vi "Set extraction scrollbar.vi"(8 "error in (no error)":errorcluster, 10 "Min frame":u32, 11 "Number of frames":u32) -> (0 "error out":errorcluster)   [LabVIEW 2017]
uses:
  Globals/gl_Time series viewer globals.vi
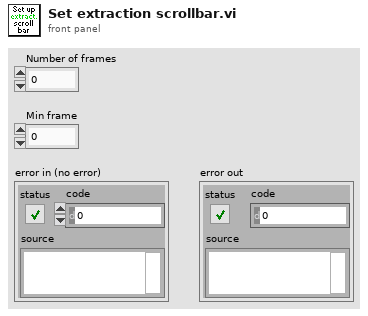
[diagram p1: front panel]
types:
  T1 = typedef "Time series viewer refs.ctl" = cluster{"This VI":refnum<vi>, "Image control":refnum<vi>, "AVI Mode ind":refnum<vi>, "Play":refnum<vi>, "Stop":refnum<vi>, "Back":refnum<vi>, "Scrollbar":refnum<vi>, "Video length info":refnum<vi>, "Expected speed values":refnum<vi>, "Intensity":refnum<vi>, "Path":refnum<vi>, "Selection sliders":refnum<vi>, "Speed Graph ref":refnum<vi>, "Frame rate set (fps)":refnum<vi>, "Channel to load":refnum<vi>, "Number of rows to generate":refnum<vi>, "Colour":refnum<vi>}
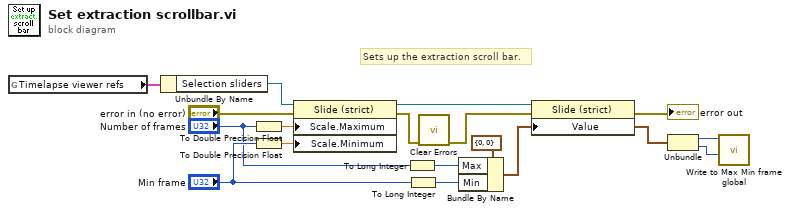
[diagram p0: block diagram]
diagram:
  # "Sets up the extraction scroll bar."
  n1 = global read "gl_Time series viewer globals.vi" "Timelapse viewer refs"() -> (w6:T1)
  n2 = Unbundle By Name(w6) -> ("Selection sliders"=w7:refnum<vi>)
  n3 = To Double Precision Float(number="Number of frames") -> (double precision float=w8:dbl)
  n4 = To Double Precision Float(number="Min frame") -> (double precision float=w16:dbl)
  n5 = property on="Property Node" class="Slide (strict)"(reference=w7, error in="error in (no error)", "Scale.Maximum"=w8, "Scale.Minimum"=w16) -> (reference out=w12:refnum<vi>, error out=w13:errorcluster)
  n6 = To Long Integer(number="Number of frames") -> (32bit integer=w3:i32)
  n7 = To Long Integer(number="Min frame") -> (32bit integer=w2:i32)
  n8 = call <vilib>:"Clear Errors.vi"("error in (no error)"=w13) -> ("error out"=w1:errorcluster)  [unwired: 5 in, 1 out]
  n9 = Bundle By Name(cluster=cluster{"Min":i32, "Max":i32} {"Min"=0, "Max"=0} ("Value"), "Max"=w3, "Min"=w2) -> (w11:cluster{"Min":i32, "Max":i32})
  n10 = property on="Property Node" class="Slide (strict)"(reference=w12, error in=w1, "Value"=w11) -> (error out=→"error out":errorcluster)  [unwired: 1 out]
  n11 = Unbundle(w11) -> ("Min"=w10:i32, "Max"=w9:i32)
  n12 = call "Write to Max Min frame global.vi"("Max cursor / End frame"=w9, "Min cursor / Start frame"=w10) -> ()  [unwired: 10 in]
